vi "SendString.vi"(8 "error in (no error)":errorcluster, 10 "String":string, 11 "TcpReader in":refnum<class "TcpReader.lvclass">) -> (0 "error out":errorcluster, 3 "TcpReader out":refnum<class "TcpReader.lvclass">)   [LabVIEW 2025, in "TcpReader.lvclass"]
doc: "Send data as a string to the TCP/IP connection"
uses:
  TcpReader.lvclass
  TcpReader.lvclass/TcpReader.ctl
  <userlib>/_OpenG.lib/error/error.llb/Filter Error Codes (Array)__ogtk.vi
  Interface/TCP/TCP/TCP.lvclass
  <userlib>/_OpenG.lib/error/error.llb/openg_error.lvlib
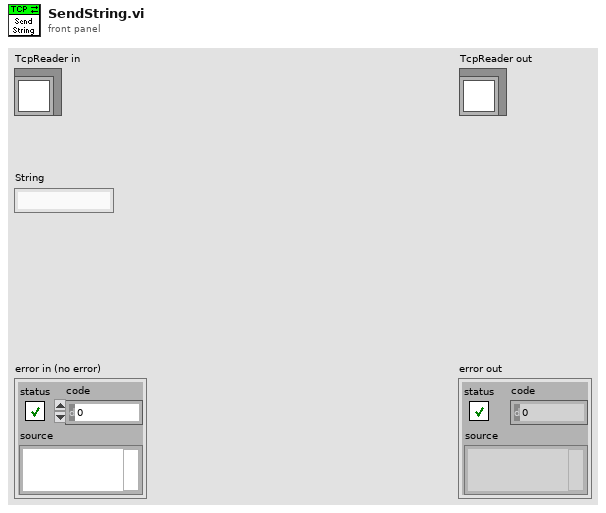
[diagram p1: front panel]
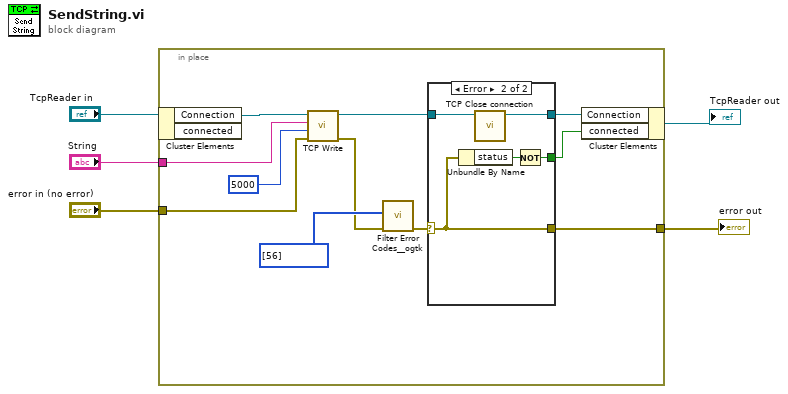
[diagram p0: block diagram]
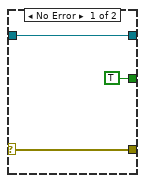
[diagram p2: hidden frame]
diagram:
  n1 = in-place "In Place Element Structure" {
    in-place-border: "String" -> [w15]
    in-place-border: "error in (no error)" -> [w13]
    in-place-border: [w7] -> w1
    n2 = in-place-cluster #1("TcpReader in") -> ("Connection"=w16:refnum<class "TCP.lvclass">)  [unwired: 1 out]
    n3 = call-dynamic "TCP Write.vi"("error in (no error)"=w13, "timeout ms (25000)"=5000, "data in"=w15, "TCP in"=w16) -> ("error out"=w10:errorcluster, "TCP out"=w9:refnum<class "TCP.lvclass">)  [unwired: 5 in, 1 out]
    n4 = call-poly <userlib>:"Filter Error Codes__ogtk.vi"("Error In"=w10, "Error Codes to Filter"=i32[] [56]) -> ("Error Out"=w11:errorcluster)  [unwired: 7 in, 2 out]
    n5 = case shown="Error" w11 {
      selector: w11 -> [w17 w20]
      tunnel: w9 -> [w18 w24]
      tunnel: [w18 w23] -> w6
      tunnel: [TRUE w21] -> w8
      tunnel: [w17 w20] -> w7
      frame No Error {
      }
      frame Error {
        n6 = Unbundle By Name(w20) -> ("status"=w22:bool)
        n7 = call-dynamic "TCP Close connection.vi"("TCP in"=w24) -> ("TCP out"=w23:refnum<class "TCP.lvclass">)  [unwired: 9 in, 1 out]
        n8 = Not(x=w22) -> (.not. x?=w21:bool)
      }
    }
    n9 = in-place-cluster #1("Connection"=w6, "connected"=w8) -> (→"TcpReader out":refnum<class "TcpReader.lvclass">)
  }
  "error out" <- w1
